vi "StopConnection.vi"(8 "ErrorIn":errorcluster, 11 "Reference":T1) -> (0 "ErrorOut":errorcluster)   [LabVIEW 2019]
uses:
  C:/Users/yasav/Downloads/prev_robocad/robocadSimLVFolder/assemblies/LibraryForLabVIEW.dll
  assemblies/LibraryForLabVIEW.dll
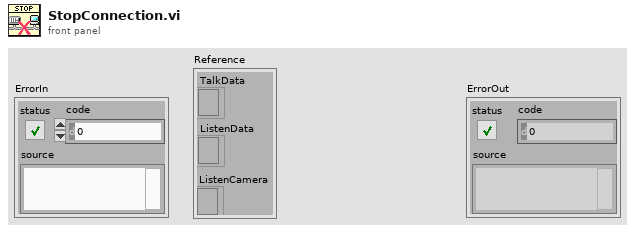
[diagram p1: front panel]
types:
  T1 = cluster{"ListenData":refnum<k24>, "ListenCamera":refnum<k24>, "TalkData":refnum<k24>}
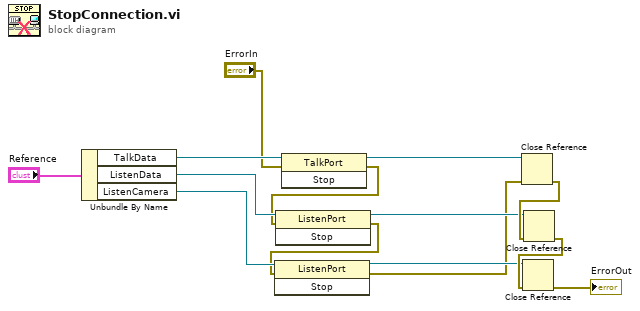
[diagram p0: block diagram]
diagram:
  n1 = Unbundle By Name("Reference") -> ("TalkData"=w6:refnum<k24>, "ListenData"=w13:refnum<k24>, "ListenCamera"=w12:refnum<k24>)
  n2 = invoke class="TalkPort" method="Stop"(reference=w6, error in="ErrorIn") -> (reference out=w4:refnum<k24>, error out=w3:errorcluster)  [unwired: 1 in, 1 out]
  n3 = invoke class="ListenPort" method="Stop"(reference=w13, error in=w3) -> (reference out=w9:refnum<k24>, error out=w11:errorcluster)  [unwired: 1 in, 1 out]
  n4 = invoke class="ListenPort" method="Stop"(reference=w12, error in=w11) -> (reference out=w7:refnum<k24>, error out=w2:errorcluster)  [unwired: 1 in, 1 out]
  n5 = Close Reference(reference=w4, error in (no error)=w2) -> (error out=w10:errorcluster)
  n6 = Close Reference(reference=w9, error in (no error)=w10) -> (error out=w8:errorcluster)
  n7 = Close Reference(reference=w7, error in (no error)=w8) -> (error out=→"ErrorOut":errorcluster)
